vi "Create directory.vi"(8 "error in (no error)":errorcluster, 10 "Directory":string, 11 "WebDAV in":refnum<class "WebDAV.lvclass">) -> (0 "error out":errorcluster, 3 "WebDAV out":refnum<class "WebDAV.lvclass">)   [LabVIEW 2015, in "RT Management.lvlib" / "WebDAV.lvclass"]
uses:
  WebDAV.lvclass
  WebDAV.lvclass/WebDAV.ctl
  Get Session.vi
  <vilib>/Utility/error.llb/Trim Whitespace.vi
  <vilib>/WebDAVClient/NI_WebDAV.lvlib
  File Transfer Behavior/File Transfer Behavior.lvclass
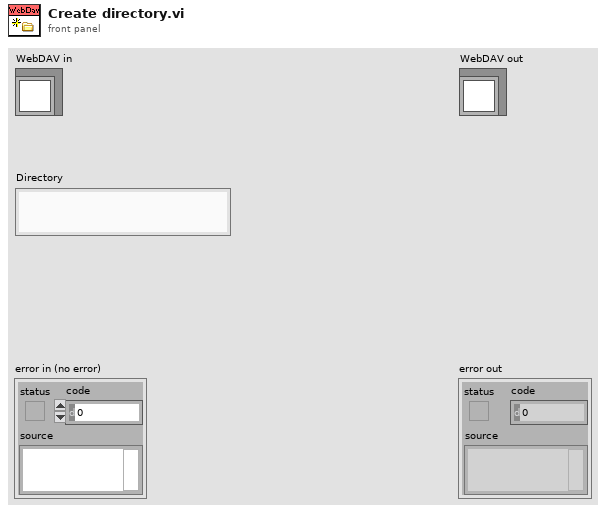
[diagram p1: front panel]
types:
  T1 = typedef "NI_WebDAV.lvlib/SessionHandle.ctl" = refnum<k1>
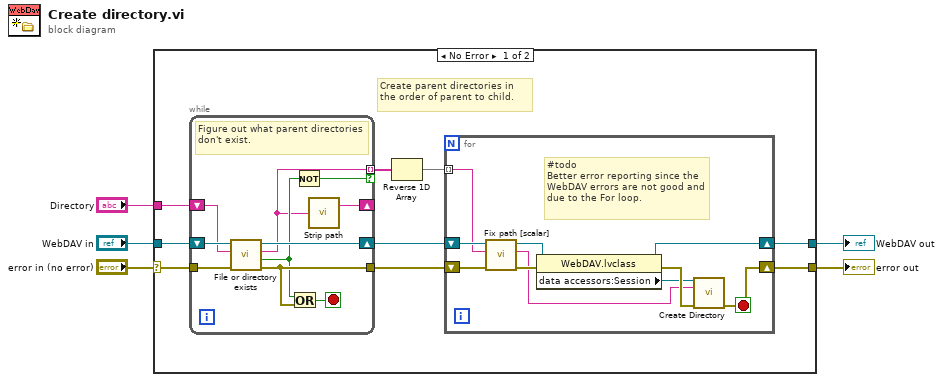
[diagram p0: block diagram]
diagram:
  n1 = case shown="No Error" "error in (no error)" {
    selector: "error in (no error)" -> [w7 w36]
    tunnel: "WebDAV in" -> [w12 w35]
    tunnel: "Directory" -> [w11 _]
    tunnel: [w6 w36] -> w4
    tunnel: [w8 w35] -> w3
    frame No Error {
      # "Create parent directories in the order of parent to child."
      n2 = while {
        tunnel: [w30] -> w13
        tunnel: w7 -> [w33]
        tunnel: [w27] -> w10 mode=indexing if=w25
        shift-right: [w26] -> _
        shift-left: w11 -> [w31]
        shift-right: [w34] -> w14
        shift-left: w12 -> [w32]
        stop <- w29 stop-if-true
        # "Figure out what parent directories don't exist."
        n3 = call-dynamic "File or directory exists.vi"("error in (no error)"=w33, "Path"=w31, "WebDAV in"=w32) -> ("error out"=w30:errorcluster, "Exists?"=w28:bool, "Path out (dup)"=w27:string, "WebDAV out"=w34:refnum<class "WebDAV.lvclass">)  [unwired: 4 in, 1 out]
        n4 = Or(x=w28, y=w30) -> (x .or. y?=w29:bool)
        n5 = Not(x=w28) -> (.not. x?=w25:bool)
        n6 = call "Strip path.vi"("Path"=w27) -> ("Stripped path"=w26:string)  [unwired: 2 in, 1 out]
      }
      n7 = Reverse 1D Array(array=w10) -> (reversed array=w9:string[])
      n8 = for {
        tunnel: w9 -> [w22] mode=indexing
        shift-right: [w16] -> w8
        shift-left: w14 -> [w24]
        shift-right: [w15] -> w6
        shift-left: w13 -> [w23]
        stop <- w15 stop-if-true
        # "#todo\nBetter error reporting since the WebDAV errors are not good and due to the For loop."
        n9 = call "Fix path [scalar].vi"("error in (no error)"=w23, "Path in"=w22, "File Transfer Behavior in"=w24) -> ("error out"=w20:errorcluster, "Path out"=w17:string, "File Transfer Behavior out"=w18:refnum<class "WebDAV.lvclass">)  [unwired: 6 in]
        n10 = property class="WebDAV.lvclass"(reference=w18, error in=w20) -> (reference out=w16:refnum<class "WebDAV.lvclass">, error out=w21:errorcluster, "data accessors:Session"=w19:T1)
        n11 = call <vilib>:"Create Directory.vi"("session handle"=w19, "relative uri"=w17, "error in (no error)"=w21) -> ("error out"=w15:errorcluster)  [unwired: 11 in, 1 out]
      }
    }
    frame Error {
    }
  }
  "error out" <- w4
  "WebDAV out" <- w3
